vi "Actividad 2. Lectura.vi"() -> ()   [LabVIEW 2020]
uses:
  <vilib>/Instr/_visa.llb/VISA Configure Serial Port (Instr).vi
panel:
  out "Boolean 3":bool
  in  "stop":bool
  out "String 3":string
  in  "String 2":string
  in  "Boolean 2":bool
  out "String":string
  in  "Boolean":bool
  in  "VISA resource name":refnum<visa-resource-name>
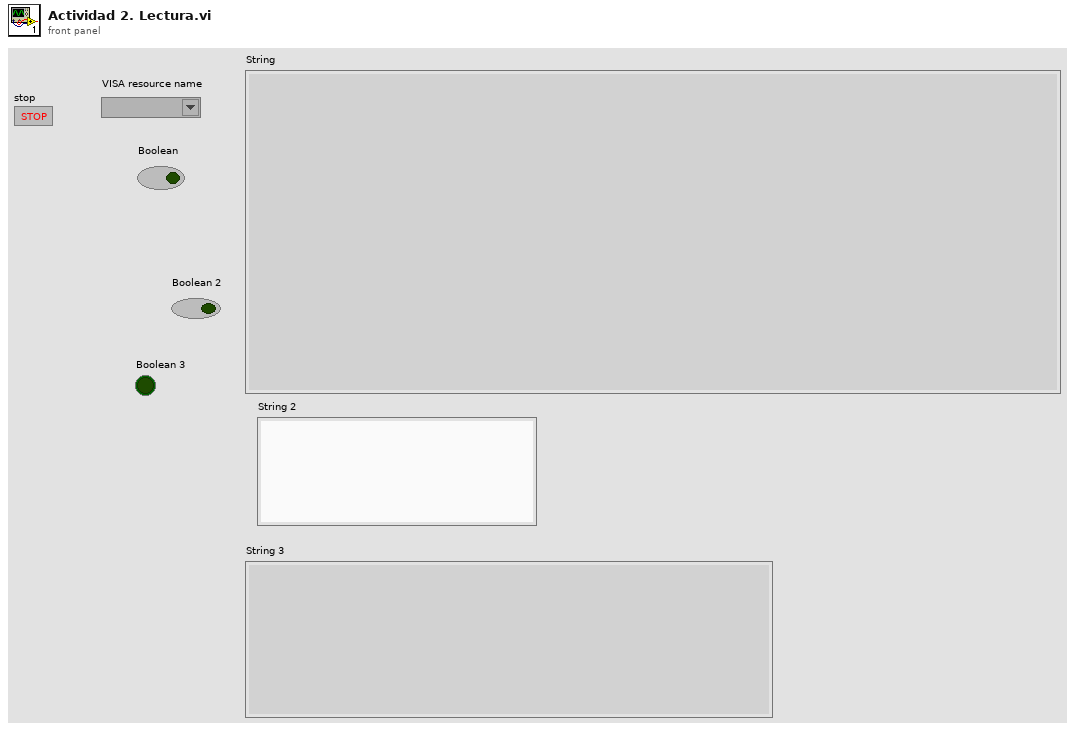
[diagram p1: front panel]
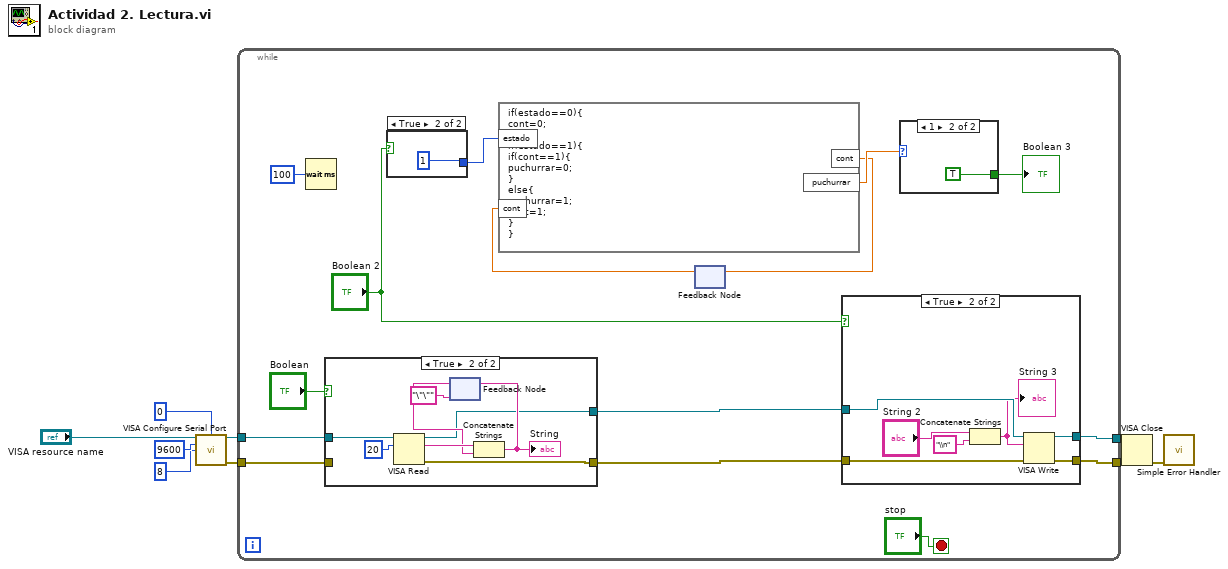
[diagram p0: block diagram]
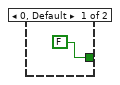
[diagram p2: hidden frame]
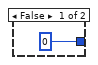
[diagram p3: hidden frame]
diagram:
  n1 = call-poly "VISA Configure Serial Port"("VISA resource name"="VISA resource name", "termination char\n(0xA = '\\n' = LF)"=u8 0 ("termination char\n(0xA = '\\n' = LF)"), "baud rate (9600)"=u32 9600, "data bits (8)"=u16 8) -> ("VISA resource name out"=w5:refnum<visa-resource-name>, "error out"=w4:errorcluster)  [unwired: 10 in]
  n2 = while {
    tunnel: w5 -> [w22]
    tunnel: w4 -> [w21]
    tunnel: [w17] -> w3
    tunnel: [w16] -> w2
    stop <- "stop" stop-if-true
    n3 = Wait (ms)(milliseconds to wait=u32 100) -> ()  [unwired: 1 out]
    n4 = case shown="True" "Boolean" {
      tunnel: w22 -> [w39 w47]
      tunnel: w21 -> [w38 _]
      tunnel: [w38 w41] -> w19
      tunnel: [w39 w40] -> w20
      frame False {
      }
      frame True {
        n5 = VISA Read(VISA resource name=w47, byte count=u32 20) -> (VISA resource name out=w40:refnum<visa-resource-name>, read buffer=w45:string, error out=w41:errorcluster)  [unwired: 1 in, 1 out]
        n6 = feedback #1("\"\"") -> (w43:string)
        n7 = Concatenate Strings(w45, w43) -> (w44:string)
        "String" <- w44
        n8 = feedback-in #1(w44) -> ()
      }
    }
    n9 = case shown="True" "Boolean 2" {
      tunnel: [0 1] -> w15
      frame False {
      }
      frame True {
      }
    }
    n10 = feedback #2() -> (w12:dbl)  [unwired: 1 in]
    n11 = formula code="if(estado==0){\ncont=0;\n}\nif(estado==1){\nif(cont==1){\npuchurrar=0;\n}\nelse{\npuchurrar=1;\ncont=1;\n}\n}"("estado"=w15, "cont"=w12) -> ("cont"=w13:dbl, "puchurrar"=w14:dbl)
    n12 = feedback-in #2(w13) -> ()
    n13 = case shown="True" "Boolean 2" {
      tunnel: w20 -> [w30 w37]
      tunnel: [w30 w36] -> w17
      tunnel: w19 -> [w29 w32]
      tunnel: [w29 w31] -> w16
      frame False {
      }
      frame True {
        n14 = Concatenate Strings("String 2", "\\n" ("string")) -> (w33:string)
        "String 3" <- w33
        n15 = VISA Write(VISA resource name=w37, write buffer=w33, error in (no error)=w32) -> (VISA resource name out=w36:refnum<visa-resource-name>, error out=w31:errorcluster)  [unwired: 1 out]
      }
    }
    n16 = case shown="1" w14 {
      tunnel: [FALSE TRUE] -> w11
      frame 0, Default {
      }
      frame 1 {
      }
    }
    "Boolean 3" <- w11
  }
  n17 = VISA Close(VISA resource name=w3, error in (no error)=w2) -> (error out=w1:errorcluster)
  n18 = call <vilib>:"Simple Error Handler.vi"("error in (no error)"=w1) -> ()  [unwired: 4 in, 5 out]
